vi "Symphony ReadWrite.vi"(0 "ServerIn":refnum<k13>, 1 "Lecture":bool=TRUE, 2 "Check Corresp":bool=TRUE, 3 "Read timeout ms(10000)":i32, 5 "ClientIn":refnum<k13>, 7 "URL":string="dstp://jandllab6.physique.usherbrooke.ca/", 9 "Message In":T1, 11 "ErrorIn (no error)":errorcluster caption="entrée d'erreur (pas d'erreur)", 12 "Écriture":bool=TRUE, 13 "CloseConn":bool) -> (4 "ServerOut":refnum<k13>, 6 "ClientOut":refnum<k13>, 10 "Data Out":T1, 15 "error out":errorcluster)   [LabVIEW 2019]
panel:
  out "Timeout":bool
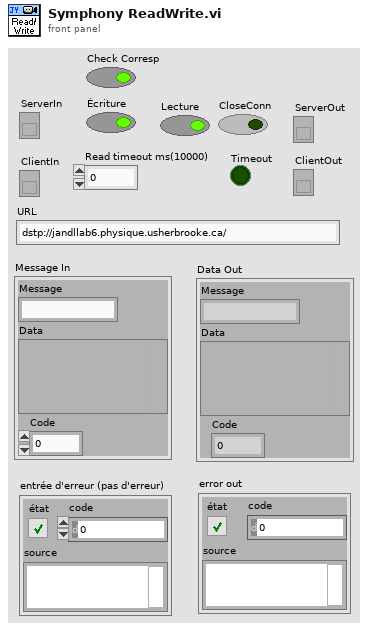
[diagram p1: front panel]
types:
  T1 = cluster{"Message":string, "Data":variant, "Code":i32}
  T2 = enum16{"Read", "Write", "ReadWrite", "BufferedRead", "BufferedReadWrite"}
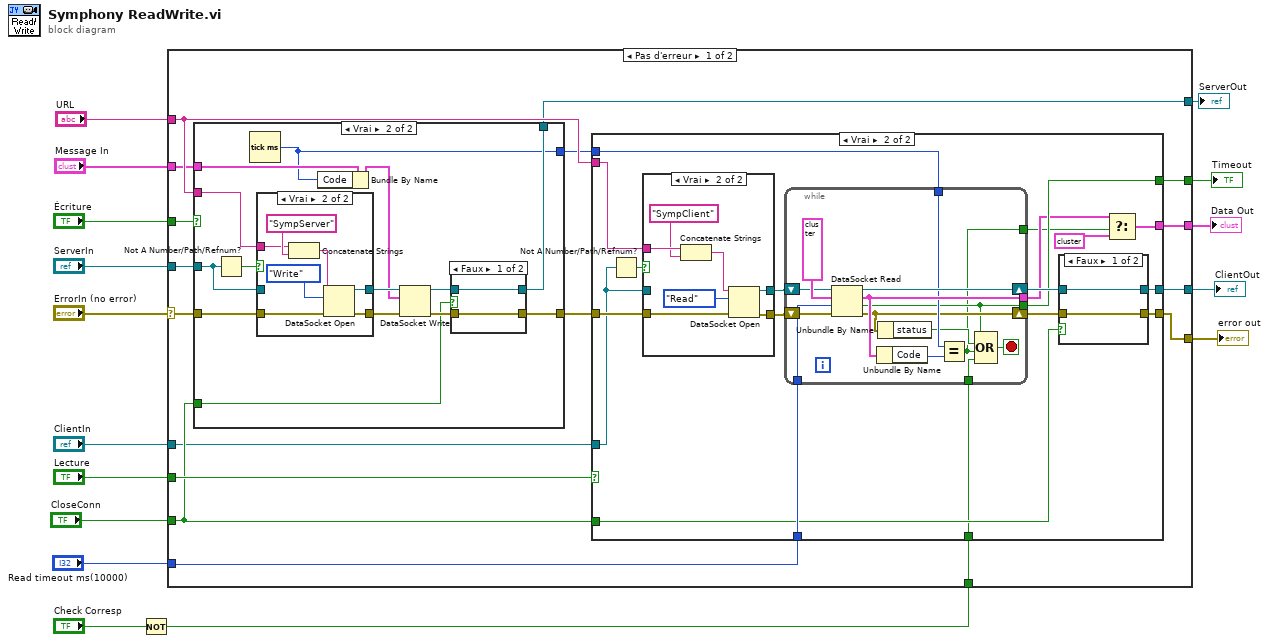
[diagram p0: block diagram]
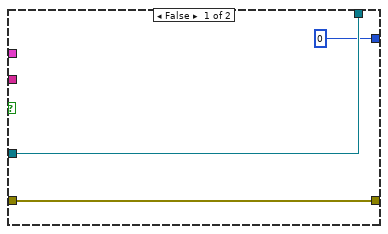
[diagram p2: hidden frame]
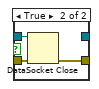
[diagram p4: hidden frame]
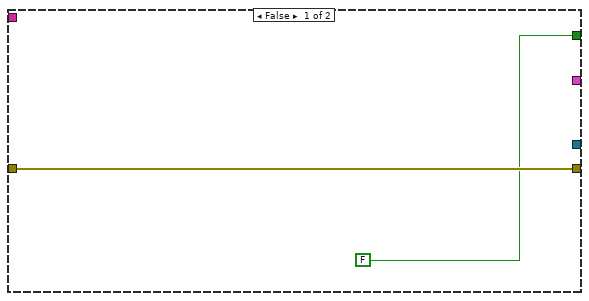
[diagram p5: hidden frame]
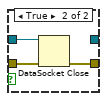
[diagram p7: hidden frame]
diagram:
  n1 = Not(x="Check Corresp") -> (.not. x?=w1:bool)
  n2 = case shown="Pas d'erreur" "ErrorIn (no error)" {
    selector: "ErrorIn (no error)" -> [w33 w114]
    tunnel: "URL" -> [w31 _]
    tunnel: "Lecture" -> [w32 _]
    tunnel: "ServerIn" -> [w29 _]
    tunnel: "CloseConn" -> [w27 _]
    tunnel: "Message In" -> [w28 _]
    tunnel: [w26 _] -> w10
    tunnel: "ClientIn" -> [w25 _]
    tunnel: [w24 _] -> w8
    tunnel: "Read timeout ms(10000)" -> [w23 _]
    tunnel: [w22 _] -> w6
    tunnel: [w21 w114] -> w5
    tunnel: "Écriture" -> [w20 _]
    tunnel: [w19 _] -> w3
    tunnel: w1 -> [w17 _]
    frame No Error {
      n3 = case shown="Vrai" w20 {
        tunnel: w33 -> [w35 w48]
        tunnel: w31 -> [_ w47]
        tunnel: [w35 w45] -> w30
        tunnel: w29 -> [w36 w42]
        tunnel: w28 -> [_ w39]
        tunnel: w27 -> [_ w41]
        tunnel: [w36 w40] -> w26
        tunnel: [u32 0 ("millisecond timer value") w37] -> w18
        frame False {
        }
        frame True {
          n4 = Not A Number/Path/Refnum?(number/path/refnum=w42) -> (NaN/Path/Refnum?=w43:bool)
          n5 = Tick Count (ms)() -> (millisecond timer value=w37:u32)
          n6 = case shown="Vrai" w43 {
            tunnel: [w51 w58] -> w50
            tunnel: [w52 w57] -> w49
            tunnel: w48 -> [w51 w56]
            tunnel: w47 -> [_ w53]
            tunnel: w42 -> [w52 _]
            frame False {
            }
            frame True {
              n7 = Concatenate Strings(w53, "SympServer") -> (w55:string)
              n8 = DataSocket Open(8:w56, 10:T2."Write" ("mode"), 11:w55) -> (0:w58:errorcluster, 3:w57:refnum<k13>)  [unwired: 1 in]
            }
          }
          n9 = Bundle By Name(cluster=w39, "Code"=w37) -> (w38:T1)
          n10 = DataSocket Write(8:w50, 10:w38, 11:w49) -> (0:w46:errorcluster, 3:w44:refnum<k13>)  [unwired: 1 in, 1 out]
          n11 = case shown="Faux" w41 {
            tunnel: w46 -> [w61 w64]
            tunnel: [w61 w63] -> w45
            tunnel: w44 -> [w60 w62]
            tunnel: [w60 _] -> w40
            frame False {
            }
            frame True {
              n12 = DataSocket Close(8:w64, 11:w62) -> (0:w63:errorcluster)  [unwired: 1 in, 1 out]
            }
          }
        }
      }
      n13 = case shown="Vrai" w32 {
        tunnel: w30 -> [w66 w85]
        tunnel: w31 -> [_ w83]
        tunnel: [w66 w80] -> w21
        tunnel: w27 -> [_ w76]
        tunnel: w25 -> [_ w78]
        tunnel: [_ w70] -> w24
        tunnel: w23 -> [_ w77]
        tunnel: [_ w74] -> w22
        tunnel: [FALSE ("timed out") w73] -> w19
        tunnel: w18 -> [_ w72]
        tunnel: w17 -> [_ w71]
        frame False {
        }
        frame True {
          n14 = Not A Number/Path/Refnum?(number/path/refnum=w78) -> (NaN/Path/Refnum?=w79:bool)
          n15 = case shown="Vrai" w79 {
            tunnel: w85 -> [w100 w108]
            tunnel: [w100 w107] -> w84
            tunnel: w83 -> [_ w106]
            tunnel: [w101 w102] -> w82
            tunnel: w78 -> [w101 _]
            frame False {
            }
            frame True {
              n16 = Concatenate Strings(w106, "SympClient") -> (w104:string)
              n17 = DataSocket Open(8:w108, 10:T2."Read" ("mode"), 11:w104) -> (0:w107:errorcluster, 3:w102:refnum<k13>)  [unwired: 1 in]
            }
          }
          n18 = while {
            tunnel: [w94] -> w69
            tunnel: w77 -> [w96]
            tunnel: [w87] -> w73
            shift-right: [w89] -> w81
            shift-left: w84 -> [w99]
            shift-right: [w95] -> w75
            shift-left: w82 -> [w97]
            tunnel: w72 -> [w92]
            tunnel: w71 -> [w90]
            tunnel: [w86] -> w68
            stop <- w91 stop-if-true
            n19 = DataSocket Read(8:w99, 9:w96, 10:T1 {"Message"="", "Data"=variant, "Code"=0}, 11:w97) -> (0:w89:errorcluster, 1:w87:bool, 2:w94:T1, 3:w95:refnum<k13>)  [unwired: 1 in, 3 out]
            n20 = Unbundle By Name(w94) -> ("Code"=w93:i32)
            n21 = Unbundle By Name(w89) -> ("status"=w88:bool)
            n22 = Equal?(x=w92, y=w93) -> (x = y?=w86:bool)
            n23 = Compound Arithmetic op=OR ("Opérateur arithmétique")(w87, w88, w86, w90) -> (w91:bool)
          }
          n24 = case shown="Faux" w76 {
            tunnel: w81 -> [w110 w113]
            tunnel: [w110 w112] -> w80
            tunnel: w75 -> [w109 w111]
            tunnel: [w109 _] -> w74
            frame False {
            }
            frame True {
              n25 = DataSocket Close(8:w113, 11:w111) -> (0:w112:errorcluster)  [unwired: 1 in, 1 out]
            }
          }
          n26 = Select(t=w69, s=w68, f=T1 {"Message"="CommError", "Data"=variant, "Code"=0} ("cas faux")) -> (s? t:f=w70:T1)
        }
      }
    }
    frame Error {
    }
  }
  "ServerOut" <- w10
  "Data Out" <- w8
  "ClientOut" <- w6
  "error out" <- w5
  "Timeout" <- w3
